vi "Robot_Cartesiano.vi"() -> ()   [LabVIEW 2021]
uses:
  <vilib>/Instr/_visa.llb/VISA Configure Serial Port (Instr).vi
panel:
  out "Direccion":string
  out "read buffer":string
  out "Pos Z":i32
  out "Pos Y":i32
  out "Pos X":i32
  in  "Mode":bool
  in  "Home Button":bool
  out "Start":bool
  out "Stop":bool
  in  "Start":bool
  in  "stop":bool
  in  "STOP":bool
  in  "Tab Control":enum32{"Autómatico", "Manual"}(tab)
  in  "EnviarAutomatico":bool
  in  "Figura":T1(ring)
  in  "Right X":bool
  in  "Left X":bool
  in  "Up Y":bool
  in  "Down Y":bool
  in  "Out Z":bool
  in  "In Z":bool
  # "Automatico"
  # "Manual"
  # "EJE Y"
  # "EJE Z"
  # "EJE X"
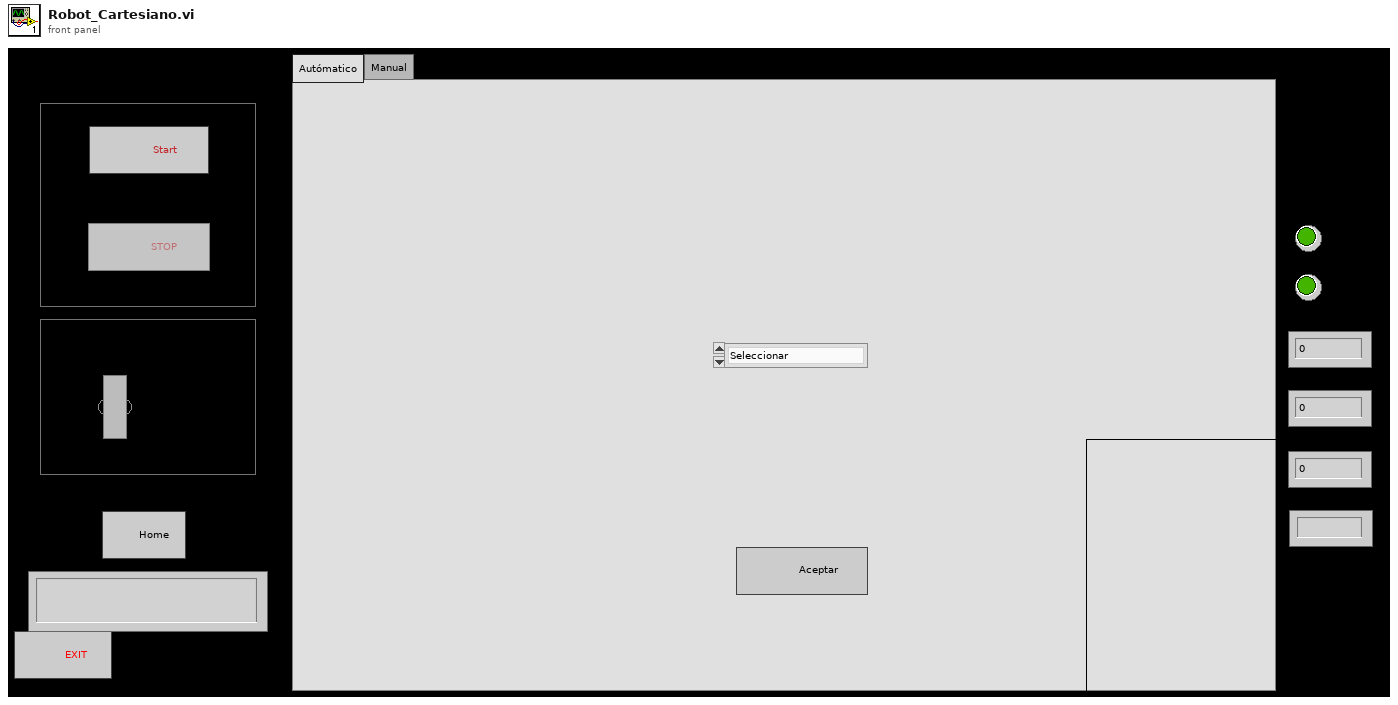
[diagram p1: front panel]
types:
  T1 = enum16{"Seleccionar", "Triangulo", "Coming soon"}
  T2 = enum8{"Enabled", "Disabled", "Disabled and Grayed Out"}
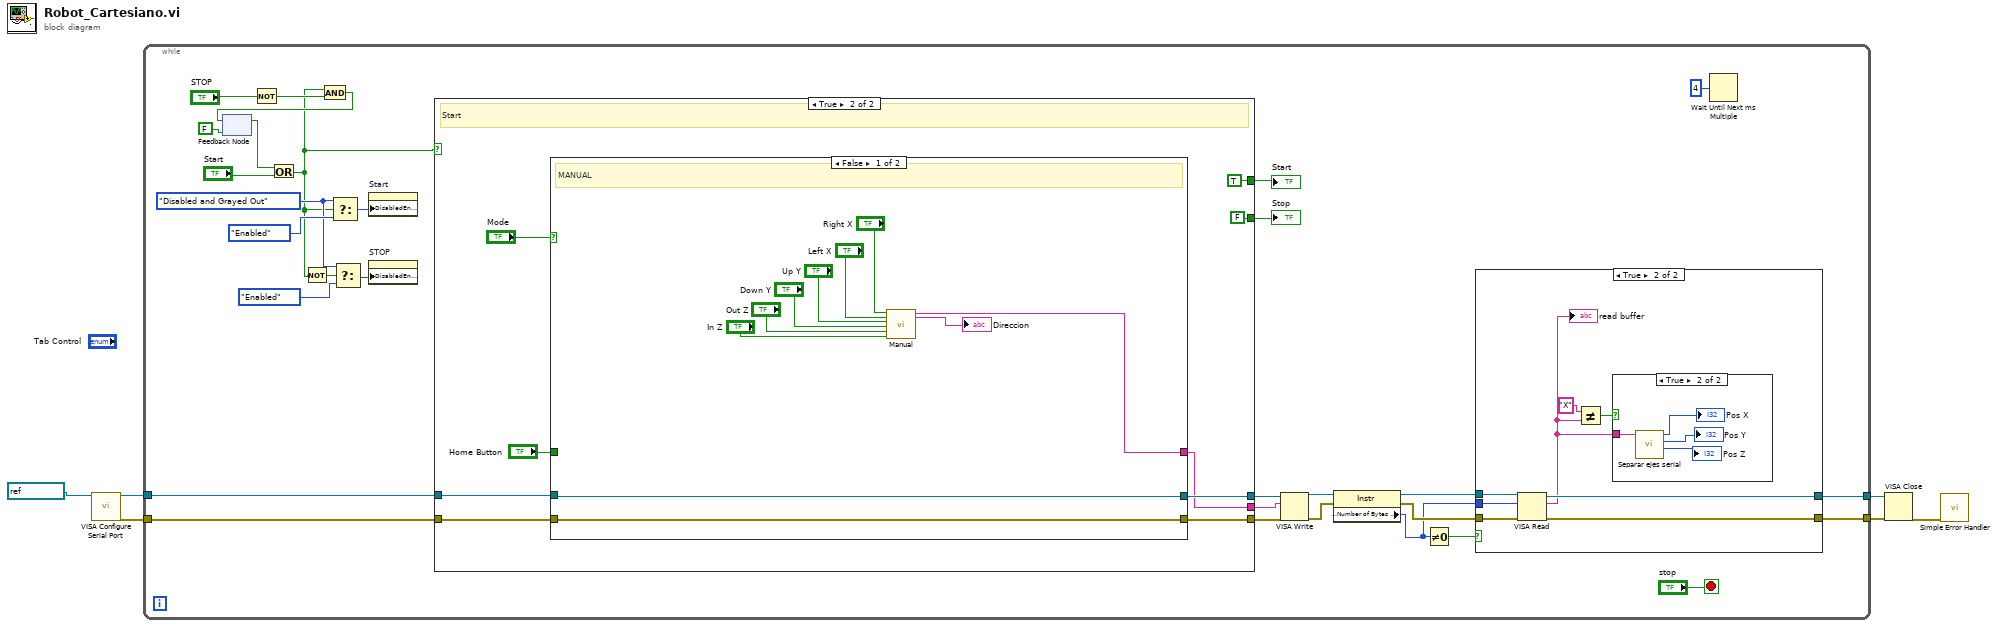
[diagram p0: block diagram]
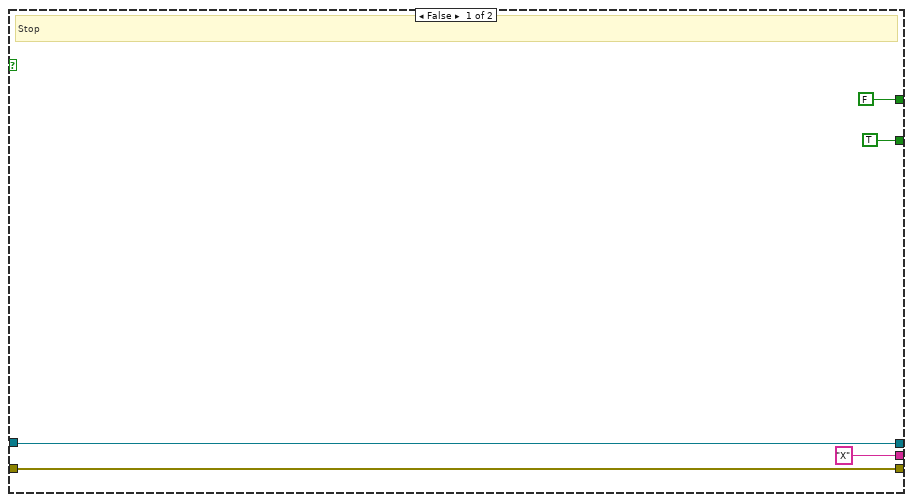
[diagram p4: hidden frame]
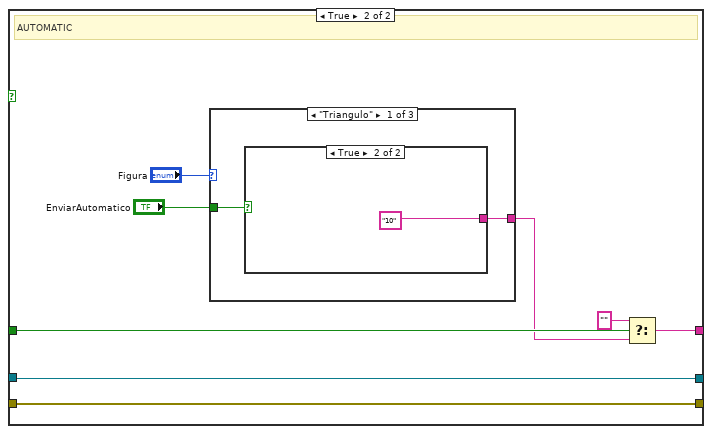
[diagram p5: hidden frame]
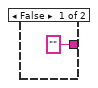
[diagram p6: hidden frame]
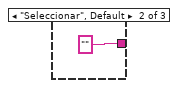
[diagram p7: hidden frame]
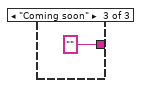
[diagram p8: hidden frame]
diagram:
  n1 = call-poly "VISA Configure Serial Port"("VISA resource name"=refnum<visa-resource-name> "COM7") -> ("VISA resource name out"=w6:refnum<visa-resource-name>, "error out"=w5:errorcluster)  [unwired: 13 in]
  n2 = while {
    tunnel: w6 -> [w19]
    tunnel: w5 -> [w18]
    tunnel: [w11] -> w2
    tunnel: [w10] -> w1
    stop <- "stop" stop-if-true
    w26 = T2."Disabled and Grayed Out" ("t")
    n3 = feedback #1(FALSE) -> (w32:bool)
    n4 = Not(x="STOP") -> (.not. x?=w34:bool)
    n5 = Or(x=w32, y="Start") -> (x .or. y?=w24:bool)
    n6 = Not(x=w24) -> (.not. x?=w25:bool)
    n7 = And(x=w24, y=w34) -> (x .and. y?=w33:bool)
    n8 = feedback-in #1(w33) -> ()
    n9 = Select(t=w26, s=w24, f=T2."Enabled" ("Disabled")) -> (s? t:f=w27:T2)
    n10 = Select(t=w26, s=w25, f=T2."Enabled") -> (s? t:f=w22:T2)
    n11 = property on="Start" class="Bool"("DisabledEnum"=w27) -> ()  [unwired: 2 in, 2 out]
    n12 = property on="STOP" class="Bool"("DisabledEnum"=w22) -> ()  [unwired: 2 in, 2 out]
    n13 = case shown="True" w24 {
      tunnel: [FALSE TRUE] -> w36
      tunnel: [TRUE FALSE] -> w35
      tunnel: ["X" w56] -> w7
      tunnel: [w52 w60] -> w20
      tunnel: w19 -> [w52 w59]
      tunnel: w18 -> [w51 w58]
      tunnel: [w51 w57] -> w17
      frame False {
        # "Stop"
      }
      frame True {
        # "Start"
        n14 = case shown="False" "Mode" {
          tunnel: [w72 w78] -> w56
          tunnel: "Home Button" -> [_ w80]
          tunnel: [w74 w76] -> w60
          tunnel: w59 -> [w74 w76]
          tunnel: w58 -> [w73 w77]
          tunnel: [w73 w77] -> w57
          frame False {
            # "MANUAL"
            n15 = call "Manual.vi"("Right X"="Right X", "Left X"="Left X", "Up Y"="Up Y", "Down Y"="Down Y", "Out Z"="Out Z", "In Z"="In Z") -> ("EnviarSerial"=w72:string, "Direccion"=→"Direccion":string)  [unwired: 12 in]
          }
          frame True {
            # "AUTOMATIC"
            n16 = case shown="\"Triangulo\"" "Figura" {
              tunnel: [w84 "" ""] -> w79
              tunnel: "EnviarAutomatico" -> [w83 _ _]
              frame "Triangulo" {
                n17 = case shown="True" w83 {
                  tunnel: ["" "10"] -> w84
                  frame False {
                  }
                  frame True {
                  }
                }
              }
              frame "Seleccionar", Default {
              }
              frame "Coming soon" {
              }
            }
            n18 = Select(t="", s=w80, f=w79) -> (s? t:f=w78:string)
          }
        }
      }
    }
    "Start" <- w36
    "Stop" <- w35
    n19 = VISA Write(VISA resource name=w20, write buffer=w7, error in (no error)=w17) -> (VISA resource name out=w13:refnum<visa-resource-name>, error out=w12:errorcluster)  [unwired: 1 out]
    n20 = property class="Instr"(reference=w13, error in=w12) -> (reference out=w16:refnum<visa-resource-name>, error out=w15:errorcluster, "Serial Settings:Number of Bytes at Serial Port"=w14:u32)
    n21 = Not Equal To 0?(x=w14) -> (x != 0?=w9:bool)
    n22 = case shown="True" w9 {
      tunnel: w16 -> [w38 w46]
      tunnel: w15 -> [w37 w45]
      tunnel: w14 -> [_ w44]
      tunnel: [w38 w43] -> w11
      tunnel: [w37 w42] -> w10
      frame False {
      }
      frame True {
        n23 = VISA Read(VISA resource name=w46, byte count=w44, error in (no error)=w45) -> (VISA resource name out=w43:refnum<visa-resource-name>, read buffer=w40:string, error out=w42:errorcluster)  [unwired: 1 out]
        "read buffer" <- w40
        n24 = Not Equal?(x="X", y=w40) -> (x != y?=w41:bool)
        n25 = case shown="True" w41 {
          tunnel: w40 -> [_ w50]
          frame False {
          }
          frame True {
            n26 = call "Separar ejes serial.vi"("Read buffer"=w50) -> ("Pos Z"=→"Pos Z":i32, "Pos Y"=→"Pos Y":i32, "Pos X"=→"Pos X":i32)  [unwired: 7 in, 1 out]
          }
        }
      }
    }
    n27 = Wait Until Next ms Multiple(millisecond multiple=u32 4) -> ()  [unwired: 1 out]
  }
  n28 = VISA Close(VISA resource name=w2, error in (no error)=w1) -> (error out=w3:errorcluster)
  n29 = call <vilib>:"Simple Error Handler.vi"("error in (no error)"=w3) -> ()  [unwired: 4 in, 5 out]
